vi "createConnection.vi"(8 "error in (no error)":errorcluster, 11 "LegacyOvenController in":refnum<class "LegacyOvenController.lvclass">) -> (0 "error out":errorcluster, 2 "IDeviceConnection":refnum<class "IDeviceConnection.lvclass">, 3 "LegacyOvenController out":refnum<class "LegacyOvenController.lvclass">)   [LabVIEW 2023, in "LegacyOvenController.lvclass"]
doc: "Factory method implementation:\nReturn a new SerialConnection object."
uses:
  LegacyOvenController.lvclass
  IDeviceConnection/IDeviceConnection.lvclass
  SerialConnection/SerialConnection.lvclass
  C:/projects/DesignPatterns_Factory/LabVIEW/FactoryMethod/IDeviceConnection/IDeviceConnection.lvclass
  LegacyOvenController.lvclass/LegacyOvenController.ctl
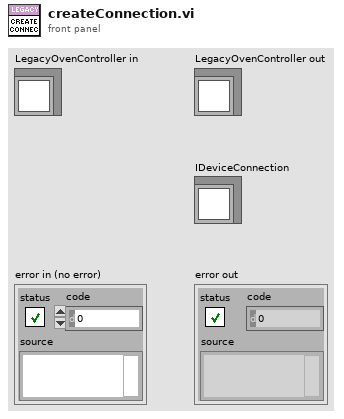
[diagram p1: front panel]
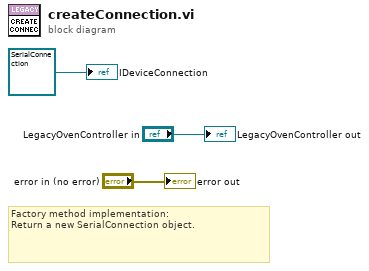
[diagram p0: block diagram]
diagram:
  # "Factory method implementation:\nReturn a new SerialConnection object."
  "error out" <- "error in (no error)"
  "LegacyOvenController out" <- "LegacyOvenController in"
  "IDeviceConnection" <- refnum<class "SerialConnection.lvclass"> refnum ("SerialConnection.lvclass")
